vi "P4CMD Convert Cfg String.vi"(7 "conversion action":T1, 8 "error in (no error)":errorcluster, 9 "configuration details in":T2, 10 "operation message":string, 11 "config data in":string) -> (0 "error out":errorcluster, 1 "config data out":string, 3 "configuration details out":T2)   [LabVIEW 2020, in "NI_SCC_P4CMD.lvlib"]
uses:
  <vilib>/SourceControl/Providers/P4CMD/NI_SCC_P4CMD.lvlib
  <vilib>/SourceControl/Providers/P4CMD/P4CMD SCC Config Info.ctl
  <vilib>/SourceControl/support/SCCSup ConfigData Conv.ctl
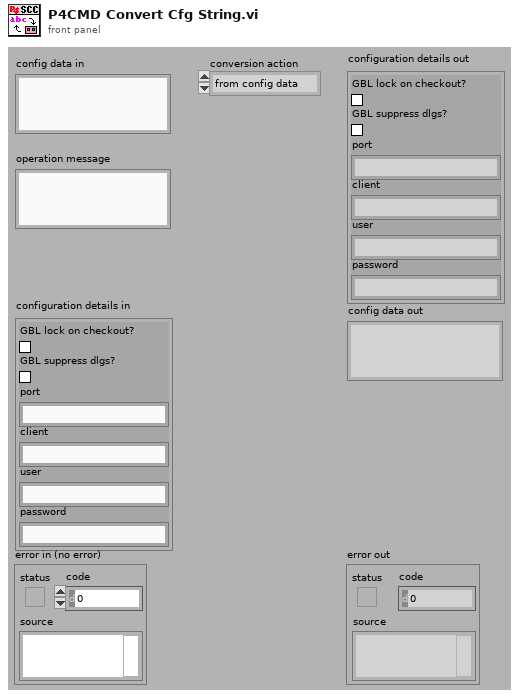
[diagram p1: front panel]
types:
  T1 = typedef "SCCSup ConfigData Conv.ctl" = enum16{"from config data", "to config data"}
  T2 = typedef "NI_SCC_P4CMD.lvlib/P4CMD SCC Config Info.ctl" = cluster{"GBL lock on checkout?":bool, "GBL suppress dlgs?":bool, "port":string, "client":string, "user":string, "password":string}
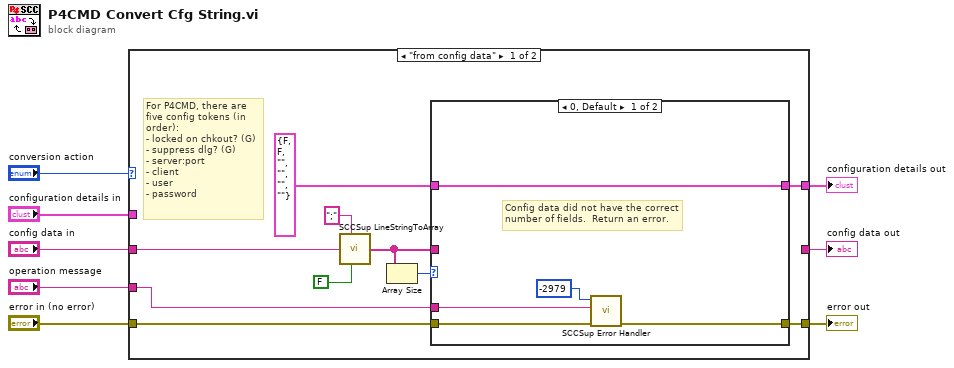
[diagram p0: block diagram]
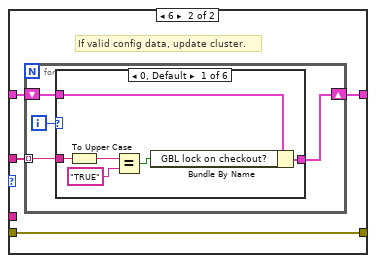
[diagram p2: hidden frame]
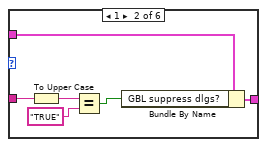
[diagram p3: hidden frame]
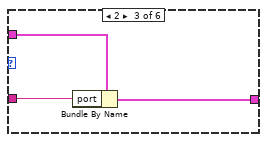
[diagram p4: hidden frame]
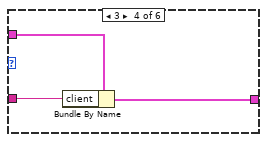
[diagram p5: hidden frame]
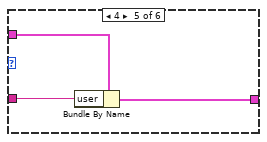
[diagram p6: hidden frame]
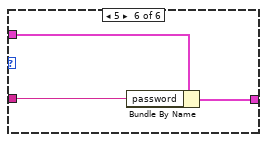
[diagram p7: hidden frame]
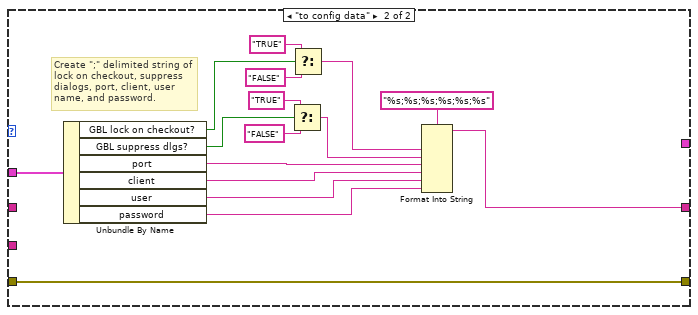
[diagram p8: hidden frame]
diagram:
  n1 = case shown="\"from config data\"" "conversion action" {
    tunnel: "config data in" -> [w15 _]
    tunnel: "configuration details in" -> [_ w71]
    tunnel: [w17 _] -> w5
    tunnel: [_ w69] -> w4
    tunnel: "error in (no error)" -> [w12 w62]
    tunnel: [w10 w62] -> w2
    tunnel: "operation message" -> [w9 _]
    frame "from config data" {
      # "For P4CMD, there are five config tokens (in order):\n- locked on chkout? (G)\n- suppress dlg? (G)\n- server:port\n- client\n- user\n- password"
      n2 = call <vilib>:"SCCSup LineStringToArray.vi"("delimiter (Tab)"=";", "line string"=w15, "remove last empty element? (T)"=FALSE) -> ("line array"=w13:string[])  [unwired: 6 in]
      n3 = Array Size(array=w13) -> (size(s)=w11:i32)
      n4 = case shown="0, Default" w11 {
        tunnel: T2 {"GBL lock on checkout?"=FALSE, "GBL suppress dlgs?"=FALSE, "port"="", "client"="", "user"="", "password"=""} ("project details in") -> [w23 w27]
        tunnel: [w23 w26] -> w17
        tunnel: w13 -> [_ w25]
        tunnel: w12 -> [w22 w24]
        tunnel: [w21 w24] -> w10
        tunnel: w9 -> [w19 _]
        frame 0, Default {
          # "Config data did not have the correct number of fields.  Return an error."
          n5 = call <vilib>:"SCCSup Error Handler.vi"("error in (no error)"=w22, "operation message"=w19, "scc error code"=-2979 ("error code")) -> ("error out"=w21:errorcluster)  [unwired: 8 in]
        }
        frame 6 {
          # "If valid config data, update cluster."
          n6 = for {
            tunnel: w25 -> [w30] mode=indexing
            shift-right: [w28] -> w26
            shift-left: w27 -> [w29]
            i -> [w31]
            n7 = case shown="0, Default" w31 {
              tunnel: w30 -> [w35 w40 w45 w48 w51 w53]
              tunnel: w29 -> [w37 w43 w46 w49 w52 w55]
              tunnel: [w36 w42 w44 w47 w50 w54] -> w28
              frame 0, Default {
                n8 = To Upper Case(1:w35) -> (0:w32:string)
                n9 = Equal?(x=w32, y="TRUE" ("format string")) -> (x = y?=w33:bool)
                n10 = Bundle By Name(cluster=w37, "GBL lock on checkout?"=w33) -> (w36:T2)
              }
              frame 1 {
                n11 = To Upper Case(1:w40) -> (0:w38:string)
                n12 = Equal?(x=w38, y="TRUE" ("format string")) -> (x = y?=w39:bool)
                n13 = Bundle By Name(cluster=w43, "GBL suppress dlgs?"=w39) -> (w42:T2)
              }
              frame 2 {
                n14 = Bundle By Name(cluster=w46, "port"=w45) -> (w44:T2)
              }
              frame 3 {
                n15 = Bundle By Name(cluster=w49, "client"=w48) -> (w47:T2)
              }
              frame 4 {
                n16 = Bundle By Name(cluster=w52, "user"=w51) -> (w50:T2)
              }
              frame 5 {
                n17 = Bundle By Name(cluster=w55, "password"=w53) -> (w54:T2)
              }
            }
          }
        }
      }
    }
    frame "to config data" {
      # "Create \";\" delimited string of lock on checkout, suppress dialogs, port, client, user name, and password."
      n18 = Unbundle By Name(w71) -> ("GBL lock on checkout?"=w66:bool, "GBL suppress dlgs?"=w56:bool, "port"=w58:string, "client"=w59:string, "user"=w60:string, "password"=w61:string)
      n19 = Select(t="TRUE" ("format string"), s=w56, f="FALSE" ("format string")) -> (s? t:f=w57:string)
      n20 = Select(t="TRUE" ("format string"), s=w66, f="FALSE" ("format string")) -> (s? t:f=w65:string)
      n21 = Format Into String(format string="%s;%s;%s;%s;%s;%s" ("delimiter (Tab)"), w65, w57, w58, w59, w60, w61) -> (resulting string=w69:string)  [unwired: 2 in, 1 out]
    }
  }
  "configuration details out" <- w5
  "config data out" <- w4
  "error out" <- w2
